vi "IVC_read.vi"(8 "error in (no error)":errorcluster, 10 "Read Pressure":bool=TRUE, 11 "VISA Refnum in":refnum<visa-resource-name>) -> (0 "error out":errorcluster, 1 "read buffer":string, 2 "IVC":string, 3 "VISA Refnum out":refnum<visa-resource-name>)   [LabVIEW 2019]
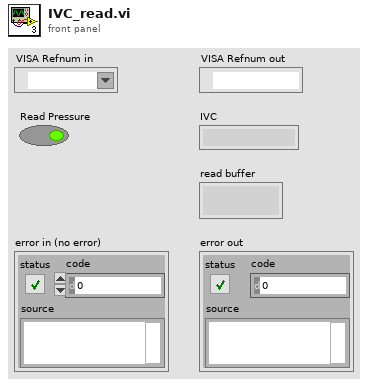
[diagram p1: front panel]
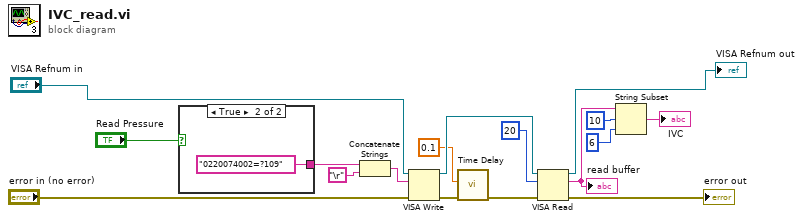
[diagram p0: block diagram]
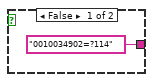
[diagram p2: hidden frame]
diagram:
  n1 = case shown="True" "Read Pressure" {
    tunnel: ["0010034902=?114" ("string") "0220074002=?109" ("string")] -> w13
    frame False {
    }
    frame True {
    }
  }
  n2 = Concatenate Strings(w13, "\r") -> (w9:string)
  n3 = VISA Write(VISA resource name="VISA Refnum in", write buffer=w9, error in (no error)="error in (no error)") -> (VISA resource name out=w6:refnum<visa-resource-name>, error out=w8:errorcluster)  [unwired: 1 out]
  n4 = call "Time Delay"("error in (no error)"=w8, "Delay Time (s)"=0.1) -> ("error out"=w3:errorcluster)  [unwired: 9 in]
  n5 = VISA Read(VISA resource name=w6, byte count=u32 20, error in (no error)=w3) -> (VISA resource name out=→"VISA Refnum out":refnum<visa-resource-name>, read buffer=w16:string, error out=→"error out":errorcluster)  [unwired: 1 out]
  "read buffer" <- w16
  n6 = String Subset(string=w16, offset (0)=10, length (rest)=6 ("length (rest)")) -> (substring=→"IVC":string)
